vi "Read Attributes.vi"(11 "Refresh Active Room Details Msg":refnum<class "Refresh Active Room Details Msg.lvclass">) -> (2 "Payload":cluster{"Active Room":string})   [LabVIEW 2023, in "Rooms Manager UI.lvlib" / "Refresh Active Room Details Msg.lvclass"]
uses:
  Refresh Active Room Details Msg.lvclass
  Refresh Active Room Details Msg.lvclass/Refresh Active Room Details Msg.ctl
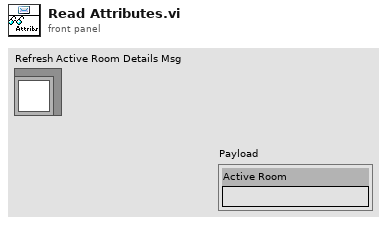
[diagram p1: front panel]
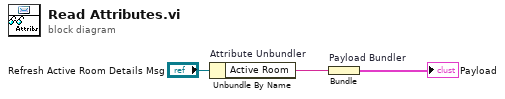
[diagram p0: block diagram]
diagram:
  n1 = Unbundle By Name "Attribute Unbundler"("Refresh Active Room Details Msg") -> ("Active Room"=w1:string)
  n2 = Bundle "Payload Bundler"("Active Room"=w1) -> (→"Payload":cluster{"Active Room":string})  [unwired: 1 in]
